vi "Get Adjusted Ring Exposure Times.vi"(10 "fptimes":sgl, 11 "inumTimes":i32) -> (2 "fptimes out":sgl, 3 "function return":u32)   [LabVIEW 2018, in "Copy of Andor SDK.lvlib"]
doc: "EXPNETTYPE unsigned int WINAPI GetAdjustedRingExposureTimes(int inumTimes, float * fptimes);"
uses:
  Copy of Andor SDK.lvlib
  <userlib>/Andor SDK/ATMCD32D.dll
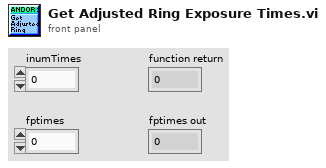
[diagram p1: front panel]
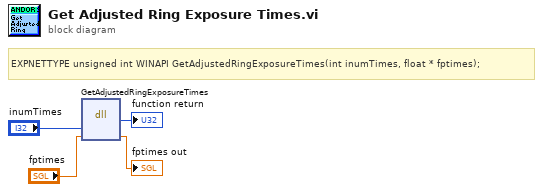
[diagram p0: block diagram]
diagram:
  # "EXPNETTYPE unsigned int WINAPI GetAdjustedRingExposureTimes(int inumTimes, float * fptimes);"
  n1 = dll-call lib="C:/Program Files (x86)/National Instruments/LabVIEW 2018/user.lib/Andor SDK/ATMCD32D.*" fn="GetAdjustedRingExposureTimes"("inumTimes"="inumTimes", "fptimes"="fptimes") -> (→"function return":u32, "fptimes"=→"fptimes out":sgl)  [unwired: 4 in, 2 out]
